vi "Delete_DVR_Occurrence.vi"(0 "Without data DVR reference":refnum<data-value>, 11 "error in (no error)":errorcluster) -> (15 "error out":errorcluster)   [LabVIEW 2020, in "Without Data.lvclass"]
doc: "This VI is used to delete the DVR created for occurrence"
uses:
  Classes/Children/Intra-Application/Children/Without data/Without Data.lvclass
  Classes/Children/Intra-Application/Children/Without data/Without Data.lvclass/Without Data.ctl
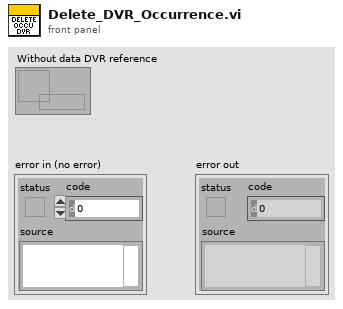
[diagram p1: front panel]
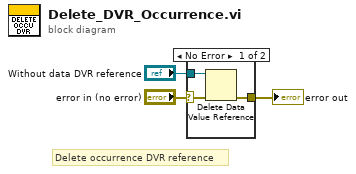
[diagram p0: block diagram]
diagram:
  # "Delete occurrence DVR reference"
  n1 = case shown="No Error" "error in (no error)" {
    selector: "error in (no error)" -> [w6 w7]
    tunnel: [w5 w7] -> w2
    tunnel: "Without data DVR reference" -> [w4 _]
    frame No Error {
      n2 = Delete Data Value Reference(data value reference=w4, error in=w6) -> (error out=w5:errorcluster)  [unwired: 1 out]
    }
    frame Error {
    }
  }
  "error out" <- w2
